vi "DSF.Engine.Plugin.Transfer.Build.vi"(8 "error in (no error)":errorcluster, 10 "Transfer":refnum<class "DSF.Engine.Transfer.lvclass">, 11 "Plugin in":refnum<class "Plugin.lvclass">) -> (0 "error out":errorcluster, 3 "Plugin out":refnum<class "Plugin.lvclass">)   [LabVIEW 2017, in "DSF.Engine.lvlib" / "Plugin.lvclass"]
uses:
  Plugin.lvclass
  Transfer/DSF.Engine.Transfer.lvclass
  Transfer/DSF.Engine.Transfer.lvclass/DSF.Engine.Transfer.ctl
  Shared/Classes/Transfer/DSF.Shared.Configuration.Transfer.lvclass/DSF.Shared.Configuration.Transfer.ctl
  Plugin.lvclass/Plugin.ctl
  Buffer/DSF.Engine.Memory.Buffer.lvclass
  Shared/Classes/Transfer/DSF.Shared.Configuration.Transfer.lvclass
  Pointer/DSF.Engine.Pointer.DBL.lvclass
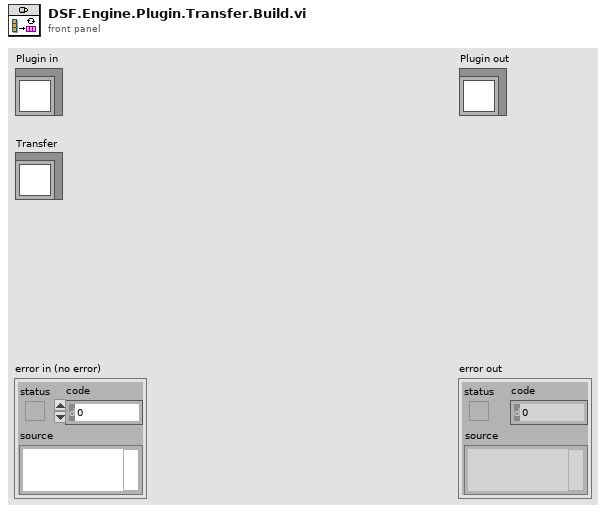
[diagram p1: front panel]
types:
  T1 = typedef "DSF.Shared.lvlib/DSF.Shared.Typedefs.Configuration.Transfer.Channel Block Descriptor.ctl" = cluster{"First Channel Descriptor":T2, "count":u64, "vs channel index":u64}
  T2 = typedef "DSF.Shared.lvlib/DSF.Shared.Typedefs.Configuration.Transfer.Channel Descriptor.ctl" = cluster{"Channel Parameters":T3, "VS Channel Ref":T5}
  T3 = typedef "DSF.Shared.lvlib/DSF.Shared.Typedefs.Configuration.Transfer.Channel Parameters.ctl" = cluster{"offset":u64, "data type":T4}
  T4 = typedef "DSF.Shared.lvlib/DSF.Shared.Typedefs.Data Type.ctl" = enum8{"Bool", "SGL", "DBL", "I8", "I16", "I32", "I64", "U8", "U16", "U32", "U64"}
  T5 = typedef "Custom Device API.lvlib/Custom Device Item Ref.ctl" = u64
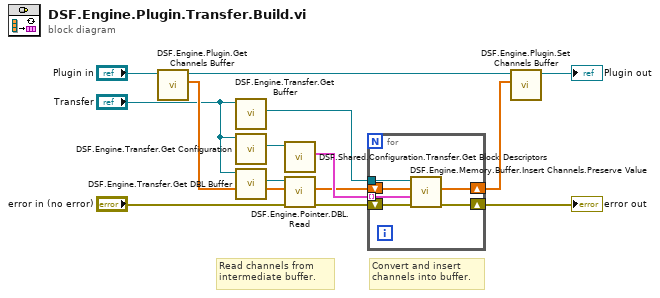
[diagram p0: block diagram]
diagram:
  # "Convert and insert channels into buffer."
  # "Read channels from intermediate buffer."
  n1 = call "DSF.Engine.Plugin.Get Channels Buffer.vi"("Plugin in"="Plugin in") -> ("channels buffer"=w3:dbl[], "Plugin out"=w5:refnum<class "Plugin.lvclass">)  [unwired: 9 in]
  n2 = call "DSF.Engine.Transfer.Get Buffer.vi"("Transfer in"="Transfer") -> ("Buffer"=w12:refnum<class "DSF.Engine.Memory.Buffer.lvclass">)  [unwired: 9 in, 1 out]
  n3 = call "DSF.Engine.Transfer.Get Configuration.vi"("Transfer in"="Transfer") -> ("Configuration"=w14:refnum<class "DSF.Shared.Configuration.Transfer.lvclass">)  [unwired: 9 in, 1 out]
  n4 = call "DSF.Engine.Transfer.Get DBL Buffer.vi"("Transfer in"="Transfer") -> ("DBL Buffer"=w10:refnum<class "DSF.Engine.Pointer.DBL.lvclass">)  [unwired: 9 in, 1 out]
  n5 = call "DSF.Shared.Configuration.Transfer.Get Block Descriptors.vi"("Transfer Configuration in"=w14) -> ("Channel Blocks"=w11:T1[])  [unwired: 9 in, 1 out]
  n6 = call "DSF.Engine.Pointer.DBL.Read.vi"("error in (no error)"="error in (no error)", "buffer in"=w3, "DBL Pointer in"=w10) -> ("error out"=w7:errorcluster, "buffer out"=w8:dbl[])  [unwired: 6 in, 1 out]
  n7 = for {
    shift-right: [w18] -> w2
    shift-left: w8 -> [w19]
    shift-right: [w17] -> w13
    shift-left: w7 -> [w20]
    tunnel: w12 -> [w16]
    tunnel: w11 -> [w15] mode=indexing
    n8 = call "DSF.Engine.Memory.Buffer.Insert Channels.Preserve Value.vi"("error in (no error)"=w20, "Channel Block"=w15, "VS Channels Array in"=w19, "Buffer in"=w16) -> ("error out"=w17:errorcluster, "VS Channels Array out"=w18:dbl[])  [unwired: 5 in, 1 out]
  }
  "error out" <- w13
  n9 = call "DSF.Engine.Plugin.Set Channels Buffer.vi"("channels buffer"=w2, "Plugin in"=w5) -> ("Plugin out"=→"Plugin out":refnum<class "Plugin.lvclass">)  [unwired: 9 in]
